vi "LJM_eReadNameString.vi"(8 "error in":errorcluster, 10 "Name":string, 11 "Handle In":i32) -> (0 "error out":errorcluster, 2 "String":string, 3 "Handle Out":i32)   [LabVIEW 2024]
uses:
  labjackm.dll
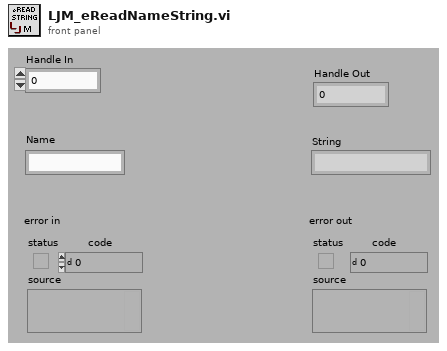
[diagram p1: front panel]
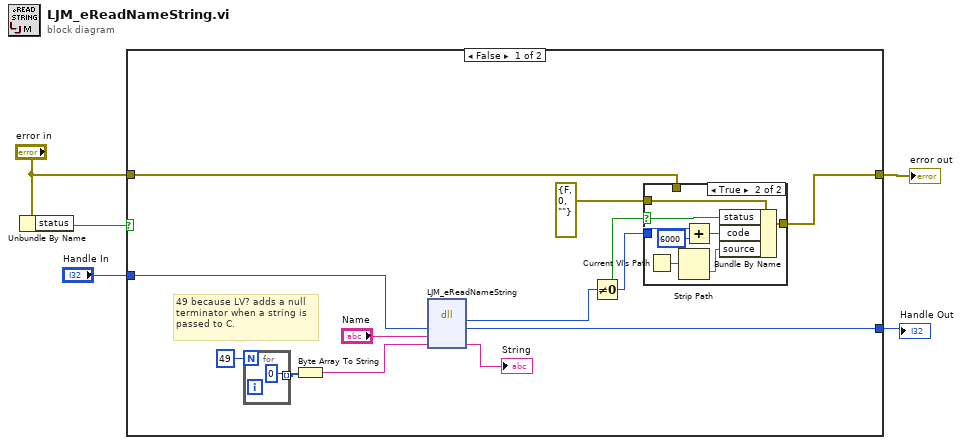
[diagram p0: block diagram]
diagram:
  n1 = Unbundle By Name("error in") -> ("status"=w5:bool)
  n2 = case shown="False" w5 {
    tunnel: "error in" -> [w14 w29]
    tunnel: [w13 w29] -> w3
    tunnel: "Handle In" -> [w11 w28]
    tunnel: [w10 w28] -> w1
    frame False {
      # "49 because LV? adds a null\nterminator when a string is\npassed to C."
      n3 = for {
        N: 49 -> [_]
        tunnel: [u8 0] -> w9 mode=indexing
      }
      n4 = Byte Array To String(unsigned byte array=w9) -> (string=w7:string)
      n5 = dll-call lib="labjackm.dll" fn="LJM_eReadNameString"("Handle"=w11, "Name"="Name", "String"=w7) -> (w17:i32, "Handle"=w10:i32, "String"=→"String":string)  [unwired: 4 in, 2 out]
      n6 = Not Equal To 0?(x=w17) -> (x != 0?=w16:bool)
      n7 = case shown="True" w16 {
        selector: w16 -> [_ w26]
        tunnel: [w19 w27] -> w13
        tunnel: errorcluster {"status"=FALSE, "code"=0, "source"=""} ("error IO") -> [_ w25]
        tunnel: w17 -> [_ w21]
        tunnel: w14 -> [w19 _]
        frame False {
        }
        frame True {
          n8 = Current VI's Path() -> (path=w23:path)
          n9 = Strip Path(path=w23) -> (name=w24:string)  [unwired: 1 out]
          n10 = Add(x=w21, y=6000) -> (x+y=w22:i32)
          n11 = Bundle By Name(cluster=w25, "status"=w26, "code"=w22, "source"=w24) -> (w27:errorcluster)
        }
      }
    }
    frame True {
    }
  }
  "error out" <- w3
  "Handle Out" <- w1
